vi "ErrorCreationType.vi"() -> ()   [LabVIEW 2018, in "ErrorCreationExecution.lvclass"]
uses:
  <userlib>/_express/CustomErrorCreator/ErrorCreationExecution/ErrorCreationExecution.lvclass
panel:
  in  "ErrorCreationType":refnum<class "ErrorCreationExecution.lvclass">
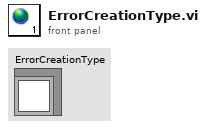
[diagram p1: front panel]
diagram:
